vi "자율주행 GPS기반 이벤트 발생.vi"() -> ()   [LabVIEW 2016]
uses:
  <vilib>/imath/engines/lvmath2/RunTimeEngine/Managers/WorkSpace/UID Generator.vi
  <vilib>/imath/engines/lvmath2/RunTimeSupport/NIMS_Error if Not Equal.vi
  <instcachedir>/0/NIMS_Error if Not Equal_43252A79AD05436189442EC0C5E5AB8A.lvgen/NIMS_Error if Not Equal_43252A79AD05436189442EC0C5E5AB8A_000.vi
  <vilib>/imath/engines/lvmath2/RunTimeEngine/IndexRead/NIMS M(S,$).vi
  <instcachedir>/0/NIMS M(S,$)_F24F360562DE41D8BE234322A2E15C65.lvgen/NIMS M(S,$)_F24F360562DE41D8BE234322A2E15C65_000.vi
  <vilib>/imath/engines/lvmath2/RunTimeEngine/RunTimeType/NIMS_RunTimeType_From StrictType (excl LVString).vi
  <instcachedir>/0/NIMS_RunTimeType_From StrictType (excl LVString)_BBF44FB49F834B71AF7A14CCEDF8BECD.lvgen/NIMS_RunTimeType_From StrictType (excl LVString)_BBF44FB49F834B71AF7A14CCEDF8BECD_000.vi
  <vilib>/imath/engines/lvmath2/RunTimeEngine/ErrorHandling/NIMS_Create Error From Enums.vi
  <vilib>/imath/engines/lvmath2/RunTimeEngine/LocalVariableDefStatement/MC_LocalVariableDefStatement_Display.vi
  <vilib>/imath/engines/lvmath2/RunTimeEngine/Managers/SymbolTable/Clear UID.vi
  <vilib>/imath/engines/lvmath2/RunTimeEngine/NodeEndStatement/NIMS_NodeEndStatement_Output.vi
  <instcachedir>/0/NIMS_NodeEndStatement_Output_53EC0D466D134D7ABD903AC30B43404B.lvgen/NIMS_NodeEndStatement_Output_53EC0D466D134D7ABD903AC30B43404B_005.vi
  <vilib>/imath/engines/lvmath2/RunTimeEngine/ErrorHandling/NIMS_Finalize Error.vi
  <vilib>/imath/engines/lvmath2/RunTimeEngine/Managers/SymbolTable/NIMS_WorkSpace.lvlib
panel:
  out "Heading angle":u16
  in  "이벤트 발생 거리(m)":dbl
  out "이벤트 발생":bool
  out "Distance":dbl
  in  "현재위치 (Lat)":dbl
  in  "현재위치 (Lon)":dbl
  out "Xn":dbl[](array[numeric])
  in  "n번째 이벤트":dbl
  in  "이벤트 예측 지점":dbl[][](array[numeric])=[[37.23256809, 126.7689735], [37.23275437, 126.7689665], [37.23288508, 126.7689025], [37.23314114, 126.7689106], [37.23328473, 126.7689497], [37.23347219, 126.7687711], [37.23339686, 126.7685929], [37.2331897, 126.7685818], [37.23310206, 126.7686283], [37.23287209, 126.7686367], [37.23277578, 126.768593], [37.23257362, 126.7685952]] format="%#.8g"
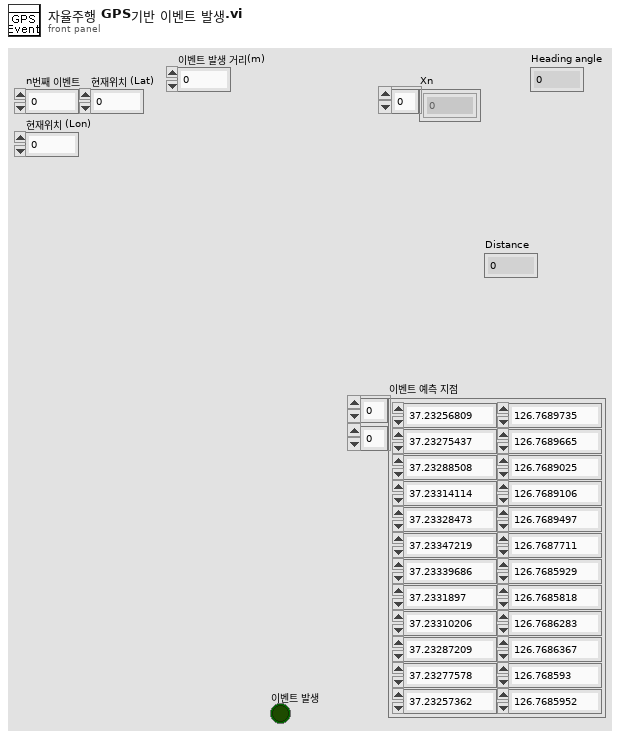
[diagram p1: front panel]
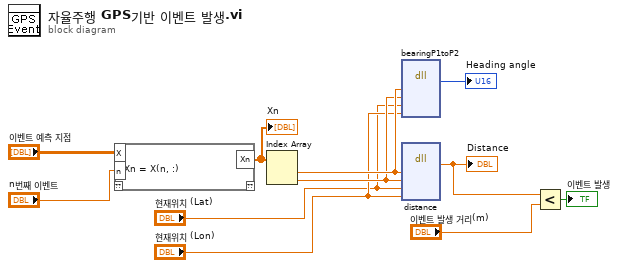
[diagram p0: block diagram]
diagram:
  n1 = mathscript code="Xn = X(n, :)"("X"="이벤트 예측 지점", "n"="n번째 이벤트") -> ("Xn"=w9:dbl[])  [unwired: 1 in, 1 out]
  "Xn" <- w9
  n2 = Index Array(array=w9) -> (element #1=w5:dbl, element #2=w4:dbl)  [unwired: 2 in]
  n3 = dll-call lib="PTH2\\abs CUsersuserDesktop[Github]_GPS Team전체프로그램DLLbearingP1toP2.dll" fn="bearingP1toP2" label="방향각"("P1_latitude"=w5, "P1_longitude"=w4, "P2_latitude"="현재위치 (Lat)", "P2_longitude"="현재위치 (Lon)") -> ("반환 타입"=→"Heading angle":u16)  [unwired: 7 in, 2 out]
  n4 = dll-call lib="PTH2aabs CUsersuserDesktop[Github]_GPS Team전체프로그램DLLdistance_of_P1toP2.dll" fn="distance" label="사이 거리"("P1_latitude"=w5, "P1_longitude"=w4, "P2_latitude"="현재위치 (Lat)", "P2_longitude"="현재위치 (Lon)") -> ("반환 타입"=w8:dbl)  [unwired: 7 in, 2 out]
  "Distance" <- w8
  n5 = Less?(x=w8, y="이벤트 발생 거리(m)") -> (x < y?=→"이벤트 발생":bool)
